vi "daqio_Get_Device_Time_Series_Data.vi"(6 "End Time":timestamp, 7 "Start Time":timestamp, 8 "error in (no error)":errorcluster, 9 "time resolution":T1, 10 "Channel Key":string, 11 "daq.io type in":T2={"daq.io ref"=refnum, "daq.io API Base"="http://dashboard.daq.io/api/v1", "Device Key"="", "Account ID"="", "online"=TRUE, "SSL"=TRUE}) -> (0 "error out":errorcluster, 2 "Datapoints out":cluster{"timestamp":timestamp, "value":dbl}[](array[cluster]), 3 "daq.io type out":T2={"daq.io ref"=refnum, "daq.io API Base"="http://dashboard.daq.io/api/v1", "Device Key"="", "Account ID"="", "online"=TRUE, "SSL"=TRUE})   [LabVIEW 2013, in "daqio minimal.lvlib"]
doc: "This VI returns all Events for a specific Device."
uses:
  daqio minimal.lvlib
  _typedefs/daqio-Type.ctl
  <vilib>/httpClient/ClientHandle.ctl
  _typedefs/daqio-rollups-resolution.ctl
  _typedefs/daqio-daily-rollups-JSON.ctl
  _typedefs/daqio-monthly-rollups-JSON.ctl
  _typedefs/daqio-hourly-rollups-JSON.ctl
  <vilib>/Easy HTTP Client/Easy HTTP.lvlib
  <vilib>/httpClient/LabVIEWHTTPClient.lvlib
panel:
  out "body":string
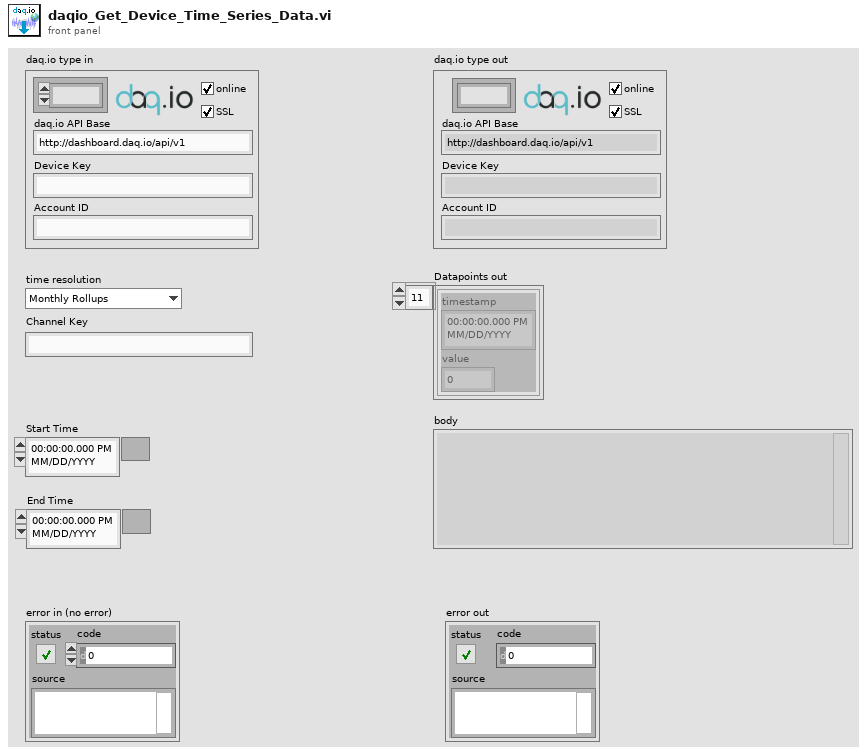
[diagram p1: front panel]
types:
  T1 = typedef "daqio minimal.lvlib/daqio-rollups-resolution.ctl" = enum16{"Monthly Rollups", "Daily Rollups", "Hourly Rollups (seconds)"}
  T2 = typedef "daqio minimal.lvlib/daqio-Type.ctl" = cluster{"daq.io ref":T3, "daq.io API Base":string, "Device Key":string, "Account ID":string, "online":bool, "SSL":bool}
  T3 = typedef "LabVIEWHTTPClient.lvlib/ClientHandle.ctl" = refnum<k1>
  T4 = typedef "daqio minimal.lvlib/daqio-daily-rollups-JSON.ctl" = cluster{"timestamp_day":string, "channel":string, "device":string, "id":string, "values":cluster{"timestamp":string, "count":i32, "max":dbl, "sum":dbl, "min":dbl}[]}
  T5 = typedef "daqio minimal.lvlib/daqio-monthly-rollups-JSON.ctl" = cluster{"timestamp_month":string, "channel":string, "device":string, "id":string, "values":cluster{"timestamp":string, "count":i32, "max":dbl, "sum":dbl, "min":dbl}[]}
  T6 = typedef "daqio minimal.lvlib/daqio-hourly-rollups-JSON.ctl" = cluster{"timestamp_hour":string, "channel":string, "device":string, "id":string, "values":dbl[]}
  T7 = cluster{"timestamp":string, "count":i32, "max":dbl, "sum":dbl, "min":dbl}[]
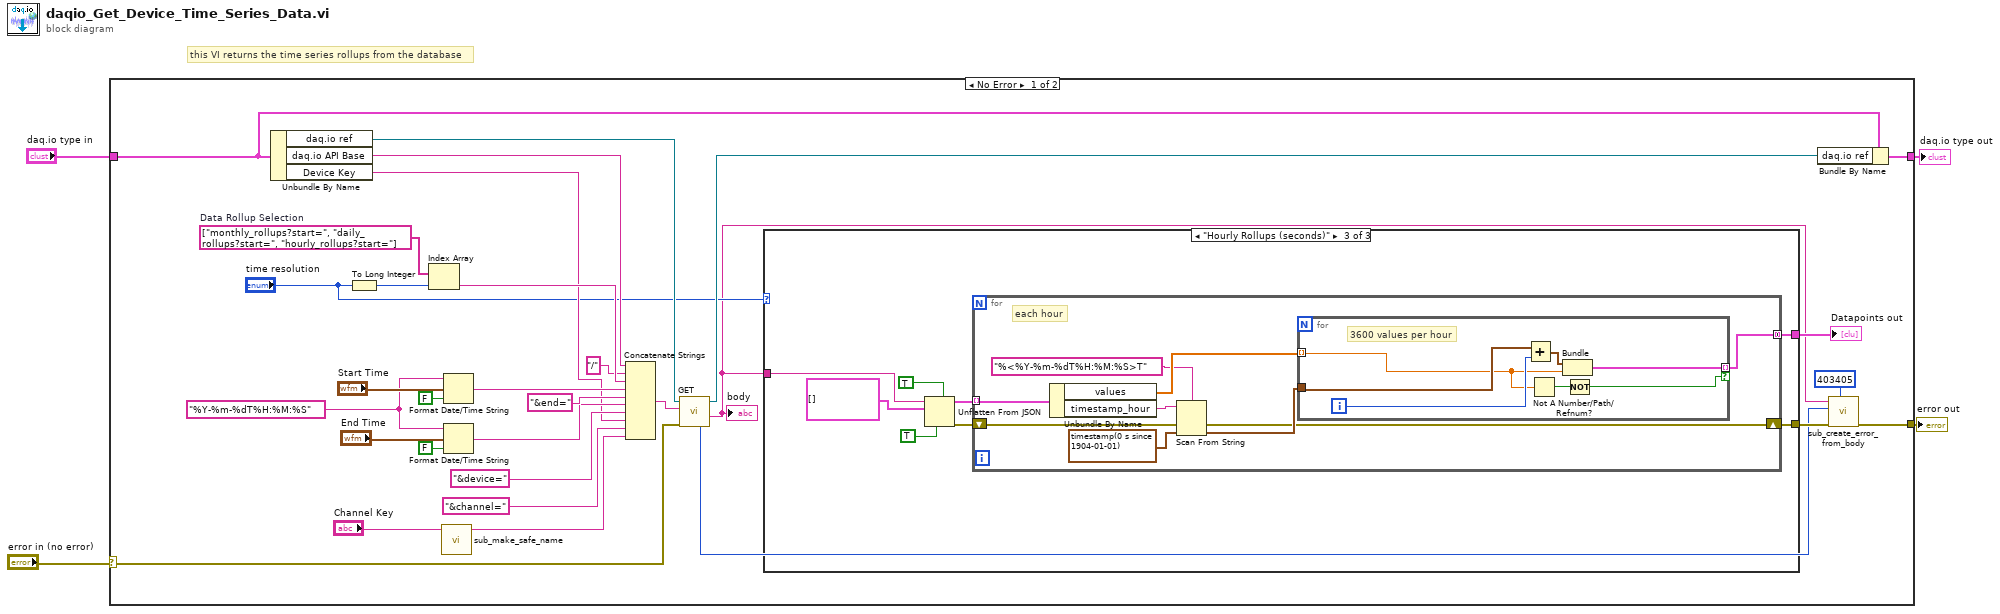
[diagram p0: block diagram]
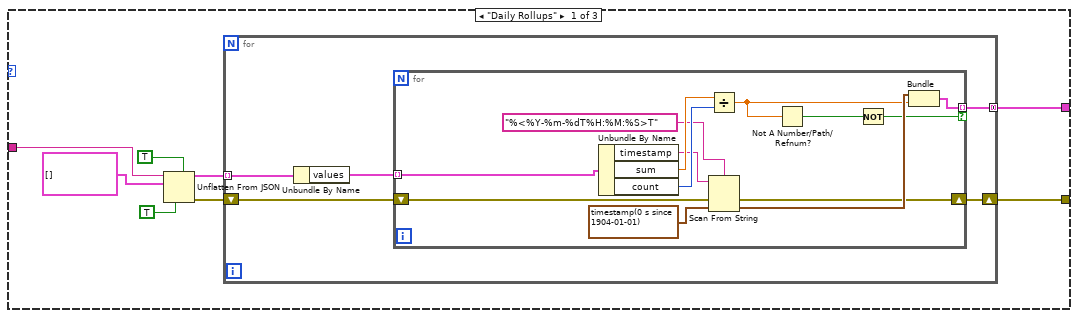
[diagram p2: hidden frame]
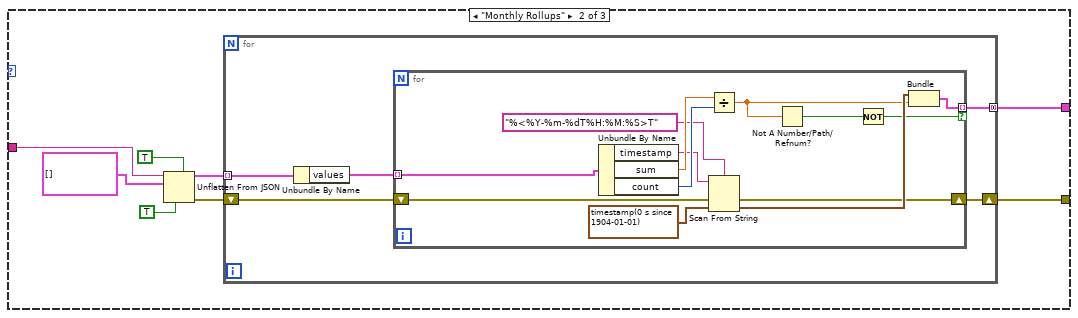
[diagram p3: hidden frame]
diagram:
  # "this VI returns the time series rollups from the database"
  n1 = case shown="No Error" "error in (no error)" {
    selector: "error in (no error)" -> [w21 w112]
    tunnel: "daq.io type in" -> [w20 w113]
    tunnel: [w35 w113] -> w3
    tunnel: [w34 w112] -> w2
    frame No Error {
      w22 = "%Y-%m-%dT%H:%M:%S" ("time format string (%c)")
      w33 = string[] ["monthly_rollups?start=", "daily_rollups?start=", "hourly_rollups?start="]  # Data Rollup Selection
      n2 = Unbundle By Name(w20) -> ("daq.io ref"=w16:T3, "daq.io API Base"=w19:string, "Device Key"=w14:string)
      n3 = To Long Integer(number="time resolution") -> (32bit integer=w7:i32)
      n4 = Index Array(array=w33, index=w7) -> (element=w32:string)
      n5 = call "sub_make_safe_name.vi"("Input String"="Channel Key") -> ("Safe Output String"=w12:string)  [unwired: 10 in]
      n6 = Format Date/Time String(time format string (%c)=w22, seconds (now)="Start Time", UTC format=FALSE) -> (date/time string=w23:string)
      n7 = Format Date/Time String(time format string (%c)=w22, seconds (now)="End Time", UTC format=FALSE) -> (date/time string=w24:string)
      n8 = Concatenate Strings(w19, "/" ("string"), w32, w23, "&end=" ("string"), w24, "&device=" ("string"), w14, "&channel=" ("string"), w12) -> (w30:string)
      n9 = call <vilib>:"GET.vi"("error in (no error)"=w21, "url"=w30, "client handle"=w16) -> ("body"=w5:string, "client handle out"=w17:T3, "HTTP Response Code"=w9:i32)  [unwired: 4 in, 2 out]
      "body" <- w5
      n10 = case shown="\"Hourly Rollups (seconds)\"" "time resolution" {
        tunnel: [w37 w63 w90] -> w11
        tunnel: w5 -> [w41 w67 w93]
        tunnel: [w39 w65 w88] -> w6
        frame "Daily Rollups" {
          n11 = Unflatten From JSON(enable LabVIEW extensions? (T)=TRUE, JSON string=w41, type and defaults=T4[] [], default null elements? (F)=TRUE) -> (value=w40:T4[], error out=w38:errorcluster)  [unwired: 3 in]
          n12 = for {
            tunnel: [w47] -> w39 mode=concatenating
            tunnel: w40 -> [w46] mode=indexing
            shift-right: [w44] -> w37
            shift-left: w38 -> [w45]
            n13 = Unbundle By Name(w46) -> ("values"=w48:T7)
            n14 = for {
              tunnel: w48 -> [w61] mode=indexing
              tunnel: [w56] -> w47 mode=indexing if=w51
              shift-right: [w49] -> w44
              shift-left: w45 -> [w50]
              n15 = Unbundle By Name(w61) -> ("timestamp"=w58:string, "sum"=w60:dbl, "count"=w59:i32)
              n16 = Divide(x=w60, y=w59) -> (x/y=w53:dbl)
              n17 = Scan From String "Scan From String"(format string="%<%Y-%m-%dT%H:%M:%S>T" ("input string"), input string=w58, error in=w50, default 1=timestamp(0 s since 1904-01-01) ("default value 1")) -> (error out=w49:errorcluster, output 1=w57:timestamp)  [unwired: 1 in, 2 out]
              n18 = Not A Number/Path/Refnum?(number/path/refnum=w53) -> (NaN/Path/Refnum?=w52:bool)
              n19 = Not(x=w52) -> (.not. x?=w51:bool)
              n20 = Bundle("default value 1"=w57, w53) -> (w56:cluster{"default value 1":timestamp, dbl})  [unwired: 1 in]
            }
          }
        }
        frame "Monthly Rollups" {
          n21 = Unflatten From JSON(enable LabVIEW extensions? (T)=TRUE, JSON string=w67, type and defaults=T5[] [], default null elements? (F)=TRUE) -> (value=w66:T5[], error out=w64:errorcluster)  [unwired: 3 in]
          n22 = for {
            tunnel: [w73] -> w65 mode=concatenating
            tunnel: w66 -> [w72] mode=indexing
            shift-right: [w70] -> w63
            shift-left: w64 -> [w71]
            n23 = Unbundle By Name(w72) -> ("values"=w74:T7)
            n24 = for {
              tunnel: w74 -> [w87] mode=indexing
              tunnel: [w82] -> w73 mode=indexing if=w77
              shift-right: [w75] -> w70
              shift-left: w71 -> [w76]
              n25 = Unbundle By Name(w87) -> ("timestamp"=w84:string, "sum"=w86:dbl, "count"=w85:i32)
              n26 = Divide(x=w86, y=w85) -> (x/y=w79:dbl)
              n27 = Scan From String "Scan From String"(format string="%<%Y-%m-%dT%H:%M:%S>T" ("input string"), input string=w84, error in=w76, default 1=timestamp(0 s since 1904-01-01) ("default value 1")) -> (error out=w75:errorcluster, output 1=w83:timestamp)  [unwired: 1 in, 2 out]
              n28 = Not A Number/Path/Refnum?(number/path/refnum=w79) -> (NaN/Path/Refnum?=w78:bool)
              n29 = Not(x=w78) -> (.not. x?=w77:bool)
              n30 = Bundle("default value 1"=w83, w79) -> (w82:cluster{"default value 1":timestamp, dbl})  [unwired: 1 in]
            }
          }
        }
        frame "Hourly Rollups (seconds)" {
          n31 = Unflatten From JSON(enable LabVIEW extensions? (T)=TRUE, JSON string=w93, type and defaults=T6[] [], default null elements? (F)=TRUE) -> (value=w92:T6[], error out=w91:errorcluster)  [unwired: 3 in]
          n32 = for {
            tunnel: w92 -> [w103] mode=indexing
            shift-right: [w97] -> w90
            shift-left: w91 -> [w99]
            tunnel: [w96] -> w88 mode=concatenating
            # "each hour"
            n33 = Unbundle By Name(w103) -> ("values"=w104:dbl[], "timestamp_hour"=w102:string)
            n34 = Scan From String "Scan From String"(format string="%<%Y-%m-%dT%H:%M:%S>T" ("input string"), input string=w102, error in=w99, default 1=timestamp(0 s since 1904-01-01) ("default value 1")) -> (error out=w97:errorcluster, output 1=w98:timestamp)  [unwired: 1 in, 2 out]
            n35 = for {
              tunnel: w104 -> [w107] mode=indexing
              tunnel: [w111] -> w96 mode=indexing if=w106
              tunnel: w98 -> [w110]
              i -> [w108]
              # "3600 values per hour"
              n36 = Add(x=w110, y=w108) -> (x+y=w109:timestamp)
              n37 = Not A Number/Path/Refnum?(number/path/refnum=w107) -> (NaN/Path/Refnum?=w105:bool)
              n38 = Bundle(w109, "seconds"=w107) -> (w111:cluster{timestamp, "seconds":dbl})  [unwired: 1 in]
              n39 = Not(x=w105) -> (.not. x?=w106:bool)
            }
          }
        }
      }
      "Datapoints out" <- w6
      n40 = Bundle By Name(cluster=w20, "daq.io ref"=w17) -> (w35:T2)
      n41 = call "sub_create_error_from_body.vi"("error code"=403405, "error in (no error)"=w11, "http code"=w9, "body"=w5) -> ("error out"=w34:errorcluster)  [unwired: 7 in]
    }
    frame Error {
    }
  }
  "error out" <- w2
  "daq.io type out" <- w3
